vi "Read Message.vi"(8 "error in (no error)":errorcluster, 11 "RemoteControl.ZMQ in":refnum<class "RemoteControl.ZMQ.lvclass">) -> (0 "error out":errorcluster, 1 "Data":string, 2 "Command":string, 3 "RemoteControl.ZMQ out":refnum<class "RemoteControl.ZMQ.lvclass">, 4 "ID":string)   [LabVIEW 2019, in "RemoteControl.ZMQ.lvclass"]
uses:
  RemoteControl.ZMQ.lvclass
  C:/Users/patrick/Documents/GitHub/Instrument-Framework/lvsrc/SMOs/RemoteControl/RemoteControl.lvclass
  RemoteControl/RemoteControl.lvclass/RemoteControl.ctl
  RemoteControl.ZMQ.lvclass/RemoteControl.ZMQ.ctl
  <vilib>/Utility/error.llb/Error Cluster From Error Code.vi
  <vilib>/ErrorRing/Error Ring.xnode
  <vilib>/addons/zeromq/zmq_socket.lvclass
  <vilib>/addons/zeromq/zmq_context.lvclass
  RemoteControl/RemoteControl.lvclass
  <userlib>/LevyLab/Instrument Framework/SMOs/JSON-RPC/JSON-RPC/JSON-RPC.lvclass
panel:
  out "Retry#":i32
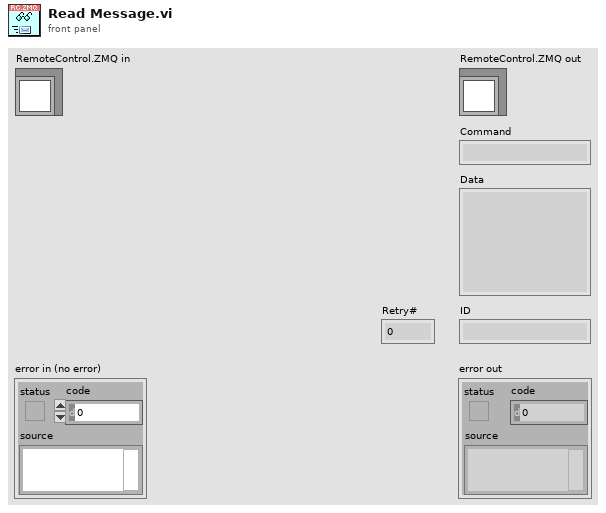
[diagram p1: front panel]
types:
  T1 = typedef "zeromq.lvlib/socket_type.ctl" = enum8{"ZMQ_PAIR", "ZMQ_PUB", "ZMQ_SUB", "ZMQ_REQ", "ZMQ_REP", "ZMQ_DEALER", "ZMQ_ROUTER", "ZMQ_PULL", "ZMQ_PUSH", "ZMQ_XPUB", "ZMQ_XSUB", "ZMQ_STREAM", "ZMQ_SERVER", "ZMQ_CLIENT", "ZMQ_RADIO", "ZMQ_DISH", "ZMQ_GATHER", "ZMQ_SCATTER", "ZMQ_DGRAM"}
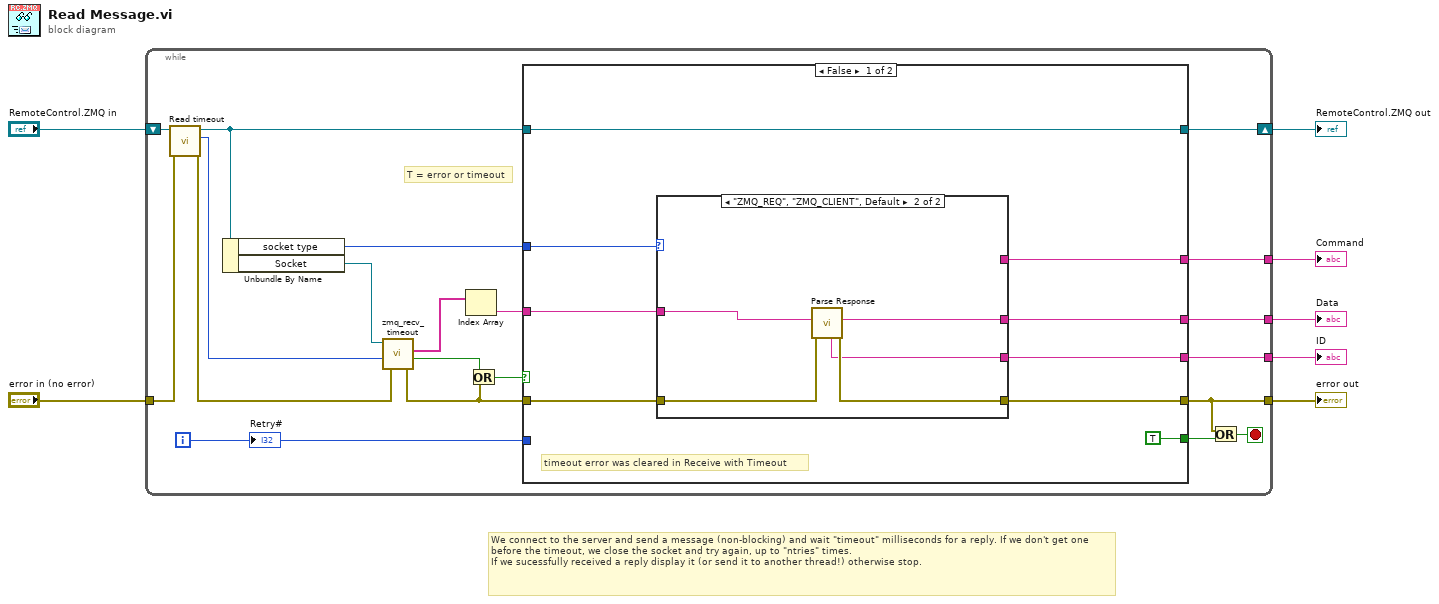
[diagram p0: block diagram]
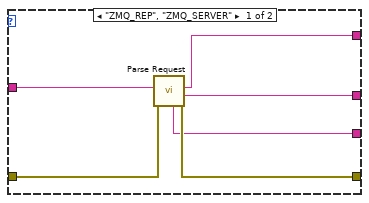
[diagram p2: hidden frame]
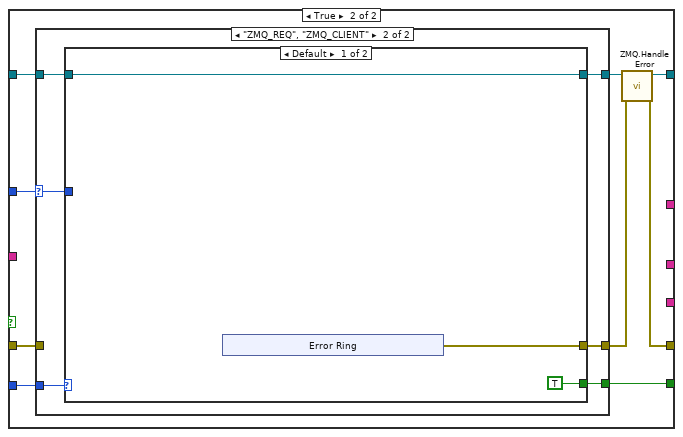
[diagram p3: hidden frame]
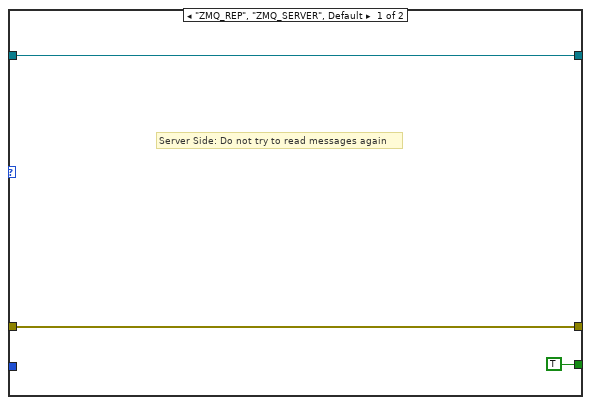
[diagram p4: hidden frame]
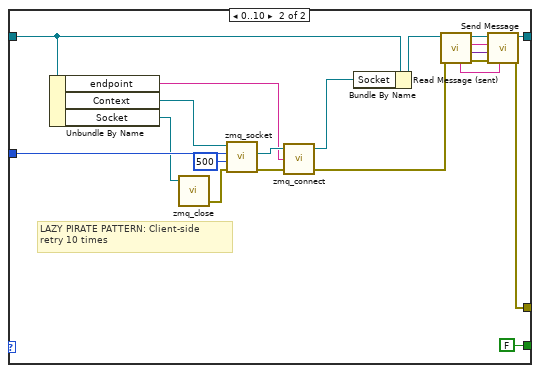
[diagram p5: hidden frame]
diagram:
  # "We connect to the server and send a message (non-blocking) and wait \"timeout\" milliseconds for a reply. If we don't get one before the timeout, we close the socket and try again, up to \"ntries\" times.\nIf we sucessfully received a reply display it (or send it to another thread!) otherwise stop."
  n1 = while {
    tunnel: [w27] -> w7
    tunnel: [w26] -> w6
    tunnel: [w25] -> w5
    tunnel: "error in (no error)" -> [w8]
    tunnel: [w11] -> w4
    shift-right: [w10] -> w3
    shift-left: "RemoteControl.ZMQ in" -> [w9]
    i -> [w20]
    stop <- w23 stop-if-true
    # "T = error or timeout"
    n2 = call "Read timeout.vi"("error in (no error)"=w8, "RemoteControl in"=w9) -> ("error out"=w14:errorcluster, "timeout"=w21:i32, "RemoteControl out"=w13:refnum<class "RemoteControl.ZMQ.lvclass">)  [unwired: 7 in]
    n3 = Unbundle By Name(w13) -> ("socket type"=w24:T1, "Socket"=w15:refnum<class "zmq_socket.lvclass">)
    n4 = call <vilib>:"zmq_recv_timeout.vi"("error in"=w14, "timeout (ms)"=w21, "socket in"=w15) -> ("error out"=w18:errorcluster, "timeout?"=w17:bool, "parts"=w12:string[])  [unwired: 1 in, 1 out]
    n5 = Index Array(array=w12) -> (element=w19:string)  [unwired: 1 in]
    n6 = Or(x=w17, y=w18) -> (x .or. y?=w16:bool)
    n7 = case shown="False" w16 {
      tunnel: [w36 _] -> w26
      tunnel: [w35 _] -> w25
      tunnel: [w34 _] -> w27
      tunnel: w24 -> [w33 w55]
      tunnel: w13 -> [w32 w56]
      tunnel: [w32 w48] -> w10
      tunnel: w20 -> [_ w54]
      tunnel: [w31 w49] -> w11
      tunnel: [TRUE w53] -> w22
      tunnel: w18 -> [w30 w52]
      tunnel: w19 -> [w28 _]
      frame False {
        # "timeout error was cleared in Receive with Timeout"
        n8 = case shown="\"ZMQ_REQ\", \"ZMQ_CLIENT\", Default" w33 {
          tunnel: w28 -> [w38 w43]
          tunnel: w30 -> [w42 w47]
          tunnel: [w41 w46] -> w31
          tunnel: [w40 _] -> w34
          tunnel: [w37 w44] -> w36
          tunnel: [w39 w45] -> w35
          frame "ZMQ_REP", "ZMQ_SERVER" {
            n9 = call <userlib>:"Parse Request.vi"("error in (no error)"=w42, "{JSON} Request"=w38) -> ("error out"=w41:errorcluster, "Params"=w37:string, "Method"=w40:string, "ID"=w39:string)  [unwired: 5 in, 1 out]
          }
          frame "ZMQ_REQ", "ZMQ_CLIENT", Default {
            n10 = call <userlib>:"Parse Response.vi"("error in (no error)"=w47, "{JSON} Response"=w43) -> ("error out"=w46:errorcluster, "results"=w44:string, "IDs"=w45:string)  [unwired: 5 in, 2 out]
          }
        }
      }
      frame True {
        n11 = case shown="\"ZMQ_REQ\", \"ZMQ_CLIENT\"" w55 {
          selector: w55 -> [_ w64]
          tunnel: w56 -> [w59 w65]
          tunnel: [w59 w63] -> w51
          tunnel: w54 -> [_ w60]
          tunnel: [w58 w62] -> w50
          tunnel: [TRUE w61] -> w53
          tunnel: w52 -> [w58 _]
          frame "ZMQ_REP", "ZMQ_SERVER", Default {
            # "Server Side: Do not try to read messages again"
          }
          frame "ZMQ_REQ", "ZMQ_CLIENT" {
            n12 = case shown="Default" w60 {
              tunnel: w65 -> [w68 w88]
              tunnel: w64 -> [_ w87]
              tunnel: [w68 w81] -> w63
              tunnel: [w67 w75] -> w62
              tunnel: [TRUE FALSE] -> w61
              frame Default {
                n13 = xnode "Error Ring"() -> ("error out"=w67:errorcluster)
              }
              frame 0..10 {
                # "LAZY PIRATE PATTERN: Client-side\nretry 10 times"
                n14 = Unbundle By Name(w88) -> ("endpoint"=w85:string, "Context"=w89:refnum<class "zmq_context.lvclass">, "Socket"=w86:refnum<class "zmq_socket.lvclass">)
                n15 = call <vilib>:"zmq_close.vi"("socket"=w86) -> ("error out"=w92:errorcluster)  [unwired: 4 in]
                n16 = call <vilib>:"zmq_socket.vi"("error in"=w92, "linger (ms)"=500, "socket type"=w87, "context in"=w89) -> ("error out"=w91:errorcluster, "socket out"=w90:refnum<class "zmq_socket.lvclass">)  [unwired: 1 in, 1 out]
                n17 = call <vilib>:"zmq_connect.vi"("error in"=w91, "endpoint"=w85, "socket in"=w90) -> ("error out"=w77:errorcluster, "socket out"=w84:refnum<class "zmq_socket.lvclass">)  [unwired: 1 in]
                n18 = Bundle By Name(cluster=w88, "Socket"=w84) -> (w83:refnum<class "RemoteControl.ZMQ.lvclass">)
                n19 = call "Read Message (sent).vi"("error in (no error)"=w77, "RemoteControl in"=w83) -> ("error out"=w78:errorcluster, "Data (Sent)"=w79:variant, "Command (Sent)"=w80:string, "RemoteControl out"=w82:refnum<class "RemoteControl.ZMQ.lvclass">, "ID (Sent)"=w76:string)  [unwired: 5 in]
                n20 = call-dynamic "Send Message.vi"("ID"=w76, "error in (no error)"=w78, "Data"=w79, "Command"=w80, "RemoteControl.ZMQ in"=w82) -> ("error out"=w75:errorcluster, "RemoteControl.ZMQ out"=w81:refnum<class "RemoteControl.ZMQ.lvclass">)  [unwired: 5 in]
              }
            }
          }
        }
        n21 = call "ZMQ.Handle Error.vi"("error in (no error)"=w50, "RemoteControl.ZMQ in"=w51) -> ("error out"=w49:errorcluster, "RemoteControl.ZMQ out"=w48:refnum<class "RemoteControl.ZMQ.lvclass">)  [unwired: 8 in]
      }
    }
    n22 = Or(x=w11, y=w22) -> (x .or. y?=w23:bool)
    "Retry#" <- w20
  }
  "error out" <- w4
  "RemoteControl.ZMQ out" <- w3
  "ID" <- w5
  "Command" <- w7
  "Data" <- w6
